vi "ChangeDoubleValue(SubVI).vi"(1 "numbers after decimal point":dbl, 2 "NumIn":dbl) -> (0 "NumOut":dbl)   [LabVIEW 2018]
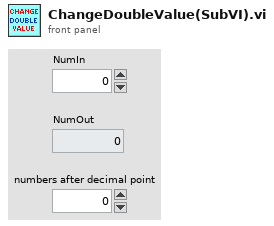
[diagram p1: front panel]
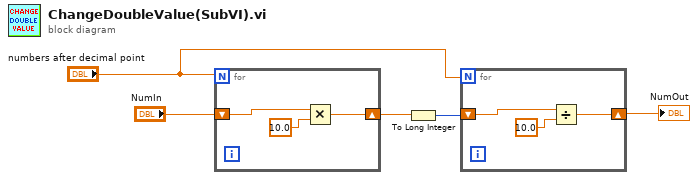
[diagram p0: block diagram]
diagram:
  n1 = for {
    N: "numbers after decimal point" -> [_]
    shift-right: [w6] -> w4
    shift-left: "NumIn" -> [w8]
    n2 = Multiply(x=w8, y=10.0) -> (x*y=w6:dbl)
  }
  n3 = To Long Integer(number=w4) -> (32bit integer=w3:i32)
  n4 = for {
    N: "numbers after decimal point" -> [_]
    shift-right: [w9] -> w1
    shift-left: w3 -> [w11]
    n5 = Divide(x=w11, y=10.0) -> (x/y=w9:dbl)
  }
  "NumOut" <- w1
